vi "UseClusterWithClass.vi"(11 "Numeric":dbl) -> (3 "ClusterWithClass":T1)   [LabVIEW 2011]
uses:
  ClassDefinitions/SimpleClassWithProperties/myClass.lvclass
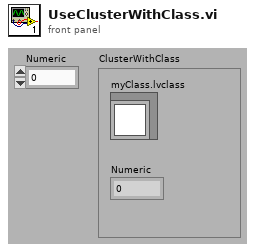
[diagram p1: front panel]
types:
  T1 = cluster{"myClass.lvclass":refnum<class "myClass.lvclass">, "Numeric":dbl}
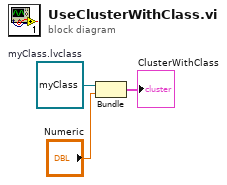
[diagram p0: block diagram]
diagram:
  w2 = refnum<class "myClass.lvclass"> refnum  # myClass.lvclass
  n1 = Bundle("myClass.lvclass"=w2, "Numeric"="Numeric") -> (→"ClusterWithClass":T1)  [unwired: 1 in]
